vi "Detected PDMs.vi"() -> (2 "PDM devices":string[](array[string]))   [LabVIEW 2021, in "audio adc shared.lvlib"]
uses:
  audio adc shared.lvlib
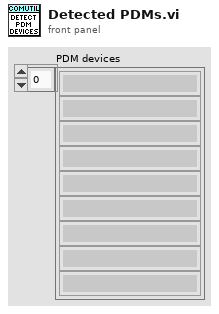
[diagram p1: front panel]
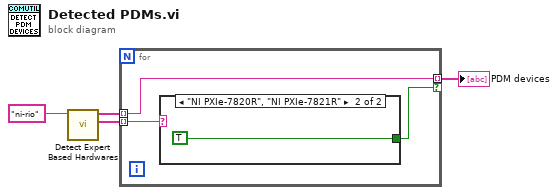
[diagram p0: block diagram]
diagram:
  n1 = call "Detect Expert Based Hardwares.vi"("Expert name"="ni-rio") -> ("Product names"=w2:string[], "Alias names"=w3:string[])  [unwired: 8 in, 1 out]
  n2 = for {
    tunnel: w3 -> [w6] mode=indexing
    tunnel: w2 -> [w7] mode=indexing
    tunnel: [w6] -> w1 mode=indexing if=w5
    n3 = case shown="\"NI PXIe-7820R\", \"NI PXIe-7821R\"" w7 {
      tunnel: [_ TRUE] -> w5
      frame "False", Default {
      }
      frame "NI PXIe-7820R", "NI PXIe-7821R" {
      }
    }
  }
  "PDM devices" <- w1
